vi "AI Regs Group UI.vi"(8 "error in (no error)":errorcluster, 11 "Node Ptr":T2 format="%.0x") -> (0 "error out":errorcluster)   [LabVIEW 2015, in "Modbus Master System Explorer.lvlib"]
uses:
  Modbus Master System Explorer.lvlib
  <vilib>/NI Veristand/Custom Device API/Custom Device Item Ref.ctl
  SubVIs/Conflict Table.ctl
  <vilib>/NI VeriStand/Custom Device API/Custom Device API.lvlib
panel:
  in  "Add One":bool
  in  "Bulk Add":bool
  out "Conflicting Input Register Mappings":T1
  in  "Header":cluster{"Section Name":string}={"Section Name"="Input Register (Analog Input) Group Settings"}
  in  "Description":string
  in  "Name":string
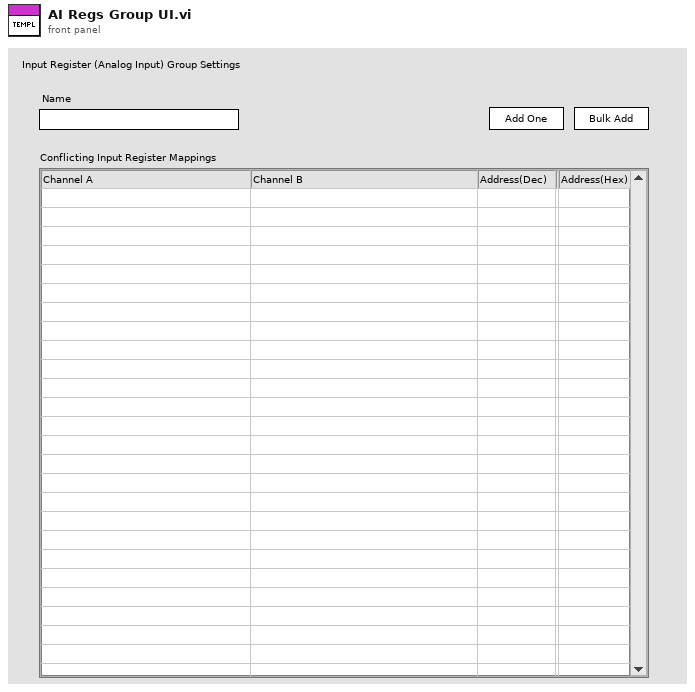
[diagram p1: front panel]
types:
  T1 = typedef "Conflict Table.ctl" = i32
  T2 = typedef "Custom Device API.lvlib/Custom Device Item Ref.ctl" = u64
  T3 = typedef "Custom Device API.lvlib/Custom Device Item Info.ctl" = cluster{"Name":string, "Is Channel":bool, "GUID":string, "Is Waveform":bool}
  T4 = cluster{"Name":string, "Name":string, "Mapping":u16}[]
  T5 = typedef "Custom Device API.lvlib/Custom Device Commands.ctl" = enum16{"Default", "Item renamed", "Shutdown", "Dynamic button pressed"}
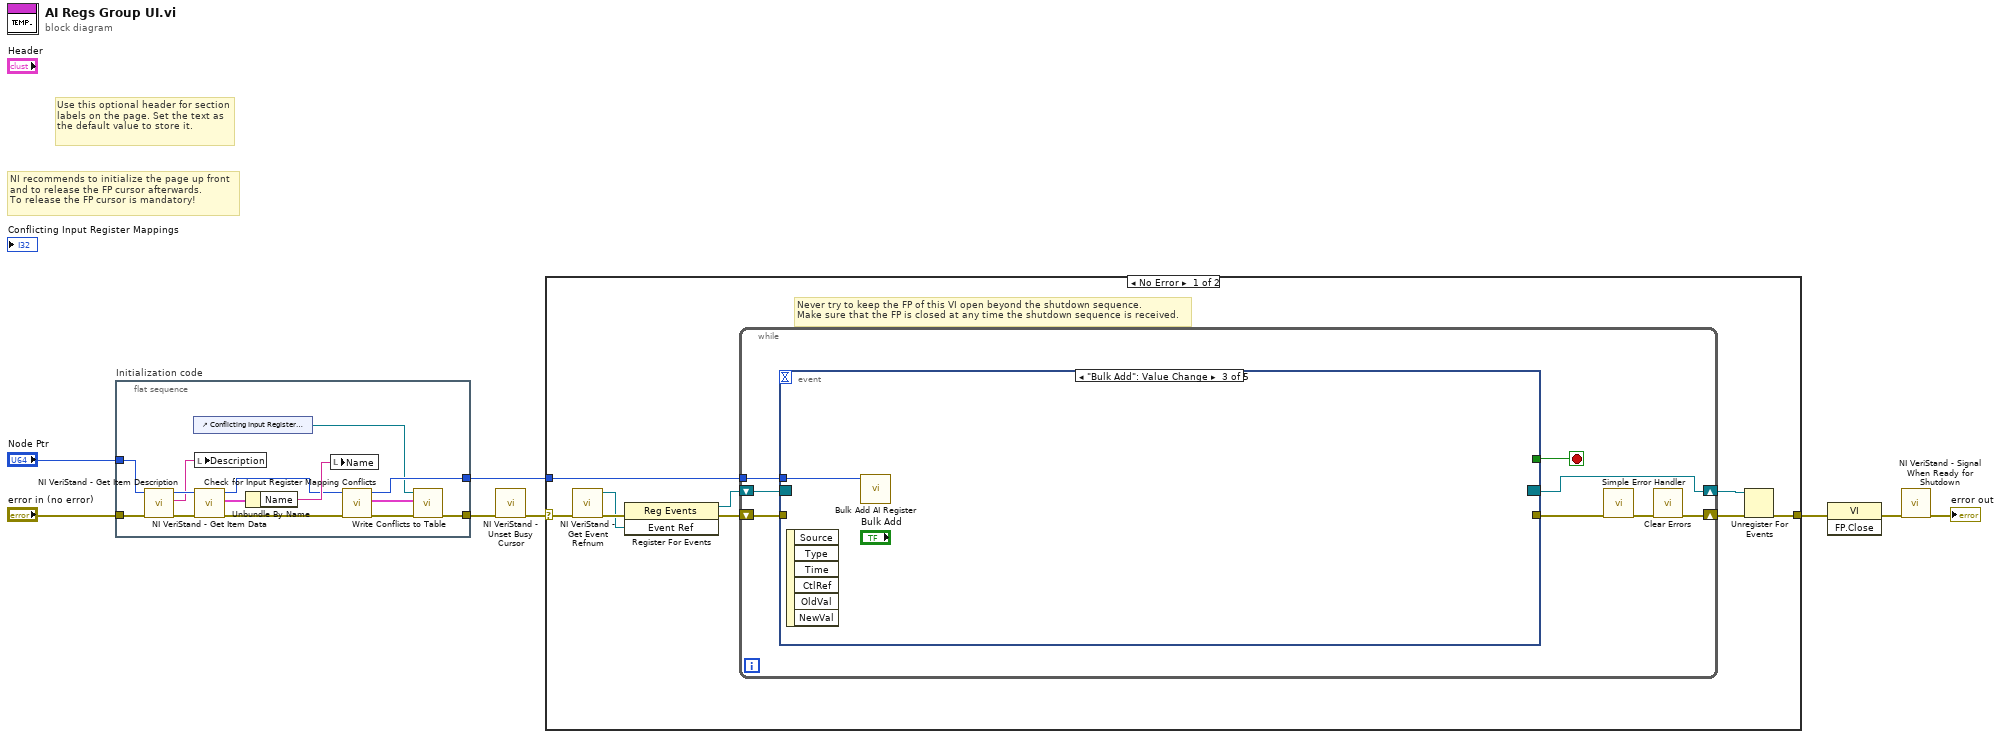
[diagram p0: block diagram]
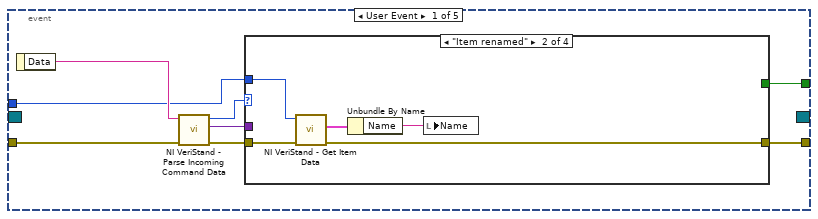
[diagram p2: hidden frame]
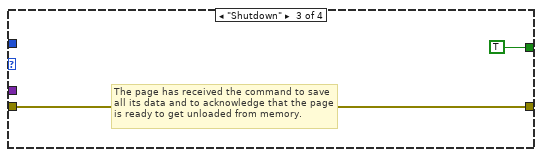
[diagram p4: hidden frame]
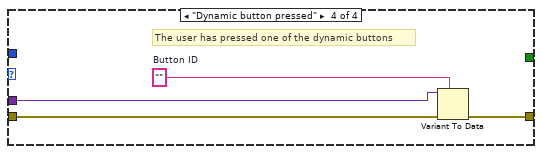
[diagram p5: hidden frame]
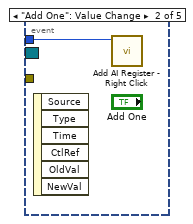
[diagram p6: hidden frame]
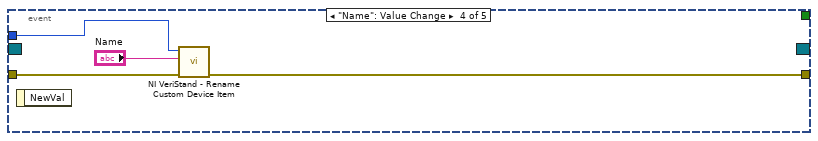
[diagram p7: hidden frame]
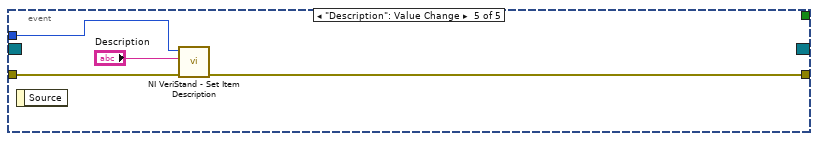
[diagram p8: hidden frame]
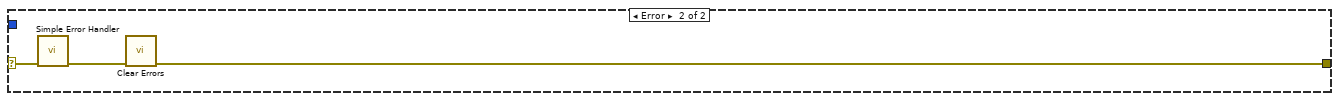
[diagram p9: hidden frame]
diagram:
  # "Use this optional header for section labels on the page. Set the text as the default value to store it."
  # "NI recommends to initialize the page up front\nand to release the FP cursor afterwards.\nTo release the FP cursor is mandatory!"
  n1 = flat-sequence "Initialization code" {
    tunnel: "error in (no error)" -> [w21]
    tunnel: "Node Ptr" -> [w20]
    tunnel: [w9] -> w4
    tunnel: [w14] -> w1
    frame #0 {
      n2 = call <vilib>:"NI VeriStand - Get Item Description.vi"("error in (no error)"=w21, "Item Ref in"=w20) -> ("error out"=w18:errorcluster, "Description"=w19:string, "Item Ref out"=w22:T2)  [unwired: 7 out]
      n3 = control-ref of="Conflicting Input Register Mappings"() -> (w12:refnum<vi>)
      n4 = local write "Description"(w19) -> ()
      n5 = call <vilib>:"NI VeriStand - Get Item Data.vi"("error in (no error)"=w18, "Item Ref in"=w22) -> ("error out"=w13:errorcluster, "Item Info"=w17:T3, "Item Ref out"=w15:T2)  [unwired: 7 out]
      n6 = Unbundle By Name(w17) -> ("Name"=w16:string)
      n7 = local write "Name"(w16) -> ()
      n8 = call "Check for Input Register Mapping Conflicts.vi"("error in (no error)"=w13, "Group Ref in"=w15) -> ("error out"=w10:errorcluster, "Conflicts"=w11:T4, "Coil Group Ref out"=w14:T2)  [unwired: 6 in, 1 out]
      n9 = call "Write Conflicts to Table.vi"("error in (no error)"=w10, "Conflicts"=w11, "MC Listbox Ref"=w12) -> ("error out"=w9:errorcluster)  [unwired: 8 in]
    }
  }
  n10 = call <vilib>:"NI VeriStand - Unset Busy Cursor.vi"("error in (no error)"=w4) -> ("error out"=w3:errorcluster)  [unwired: 10 out]
  n11 = case shown="No Error" w3 {
    selector: w3 -> [w23 w72]
    tunnel: [w28 w70] -> w8
    tunnel: w1 -> [w24 _]
    frame No Error {
      # "Never try to keep the FP of this VI open beyond the shutdown sequence.\nMake sure that the FP is closed at any time the shutdown sequence is received."
      n12 = call <vilib>:"NI VeriStand - Get Event Refnum.vi"("error in (no error)"=w23) -> ("error out"=w31:errorcluster, "Event Ref"=w27:refnum<user-event>)  [unwired: 9 out]
      n13 = register-events(error in=w31, w27) -> (reference out=w25:refnum<event-registration>, error out=w26:errorcluster)  [unwired: 1 in]
      n14 = while {
        tunnel: w24 -> [w35]
        shift-right: [w32] -> w29
        shift-left: w26 -> [w38]
        shift-right: [w39] -> w30
        shift-left: w25 -> [w37]
        stop <- w36 stop-if-true
        n15 = event shown="[2] \"Bulk Add\": Value Change" {
          selector: w37 -> [_ _ _ _ _]
          dyn-events: [_ _ _ _ _] -> w39
          timeout: _ -> [_ _ _ _ _]
          tunnel: w38 -> [w47 _ _ w65 w68]
          tunnel: [w43 _ _ _ _] -> w36
          tunnel: [w42 _ _ w64 w67] -> w34
          tunnel: w35 -> [w41 w60 w61 w63 w69]
          event User Event {
            n16 = event-data() -> ("Data"=w46:string)  [unwired: 1 out]
            n17 = call <vilib>:"NI VeriStand - Parse Incoming Command Data.vi"("error in (no error)"=w47, "Incoming data"=w46) -> ("error out"=w45:errorcluster, "Outgoing data"=w40:variant, "Action"=w44:T5)  [unwired: 7 out]
            n18 = case shown="\"Item renamed\"" w44 {
              tunnel: w45 -> [w48 w53 w54 w59]
              tunnel: [_ _ TRUE _] -> w43
              tunnel: [w48 w50 w54 w56] -> w42
              tunnel: w41 -> [_ w52 _ _]
              tunnel: w40 -> [_ _ _ w58]
              frame "Default", Default {
              }
              frame "Item renamed" {
                n19 = call <vilib>:"NI VeriStand - Get Item Data.vi"("error in (no error)"=w53, "Item Ref in"=w52) -> ("error out"=w50:errorcluster, "Item Info"=w51:T3)  [unwired: 8 out]
                n20 = Unbundle By Name(w51) -> ("Name"=w49:string)
                n21 = local write "Name"(w49) -> ()
              }
              frame "Shutdown" {
                # "The page has received the command to save all its data and to acknowledge that the page is ready to get unloaded from memory."
              }
              frame "Dynamic button pressed" {
                w57 = ""  # Button ID
                # "The user has pressed one of the dynamic buttons"
                n22 = Variant To Data(error in=w59, type=w57, Variant=w58) -> (error out=w56:errorcluster)  [unwired: 1 out]
              }
            }
          }
          event "Add One": Value Change {
            n23 = event-data() -> ()  [unwired: 7 out]
            n24 = call "Add AI Register - Right Click.vi"("Node Ptr"=w60) -> ()  [unwired: 11 in]
          }
          event "Bulk Add": Value Change {
            n25 = event-data() -> ()  [unwired: 7 out]
            n26 = call "Bulk Add AI Register.vi"("Node Ptr"=w61) -> ()  [unwired: 11 in]
          }
          event "Name": Value Change {
            n27 = event-data() -> ()  [unwired: 2 out]
            n28 = call <vilib>:"NI VeriStand - Rename Custom Device Item.vi"("error in (no error)"=w65, "New Name"="Name", "Item Ref in"=w63) -> ("error out"=w64:errorcluster)  [unwired: 1 in, 7 out]
          }
          event "Description": Value Change {
            n29 = event-data() -> ()  [unwired: 2 out]
            n30 = call <vilib>:"NI VeriStand - Set Item Description.vi"("error in (no error)"=w68, "Description"="Description", "Item Ref in"=w69) -> ("error out"=w67:errorcluster)  [unwired: 8 out]
          }
        }
        n31 = call <vilib>:"Simple Error Handler.vi"("error in (no error)"=w34) -> ("error out"=w33:errorcluster)  [unwired: 1 in, 7 out]
        n32 = call <vilib>:"Clear Errors.vi"("error in (no error)"=w33) -> ("error out"=w32:errorcluster)  [unwired: 1 in, 5 out]
      }
      n33 = Unregister For Events(event registration refnum=w30, error in=w29) -> (error out=w28:errorcluster)
    }
    frame Error {
      n34 = call <vilib>:"Simple Error Handler.vi"("error in (no error)"=w72) -> ("error out"=w71:errorcluster)  [unwired: 1 in, 7 out]
      n35 = call <vilib>:"Clear Errors.vi"("error in (no error)"=w71) -> ("error out"=w70:errorcluster)  [unwired: 1 in, 5 out]
    }
  }
  n36 = invoke class="VI" method="FP.Close"(error in=w8) -> (error out=w7:errorcluster)  [unwired: 2 in, 2 out]
  n37 = call <vilib>:"NI VeriStand - Signal When Ready for Shutdown.vi"("error in (no error)"=w7) -> ("error out"=→"error out":errorcluster)  [unwired: 10 out]
